vi "Status Update.vi"(8 "error in (no error)":errorcluster, 9 "Status":string, 10 "Name":string, 11 "Server in":refnum<class "Server.lvclass">) -> (0 "error out":errorcluster, 3 "Server out":refnum<class "Server.lvclass">)   [LabVIEW 2020, in "Server.lvlib" / "Server.lvclass"]
uses:
  Server.lvclass
  Server.lvclass/Server.ctl
  Chat Window Model/Chat Window Model Messages/Update Status Log Msg/Update Status Log Msg.lvclass/Update Status Log Msg.ctl
  <vilib>/ActorFramework/Message Enqueuer/Message Enqueuer.lvclass/Message Enqueuer.ctl
  <vilib>/ActorFramework/Message Enqueuer/Enqueue.vi
  Chat Window Model/Chat Window Model Messages/Update Status Log Msg/Update Status Log Msg.lvclass
  C:/Program Files/National Instruments/LabVIEW 2020/vi.lib/ActorFramework/Message/Message.lvclass
  <vilib>/ActorFramework/Message Priority Queue/Priority Enqueue.vi
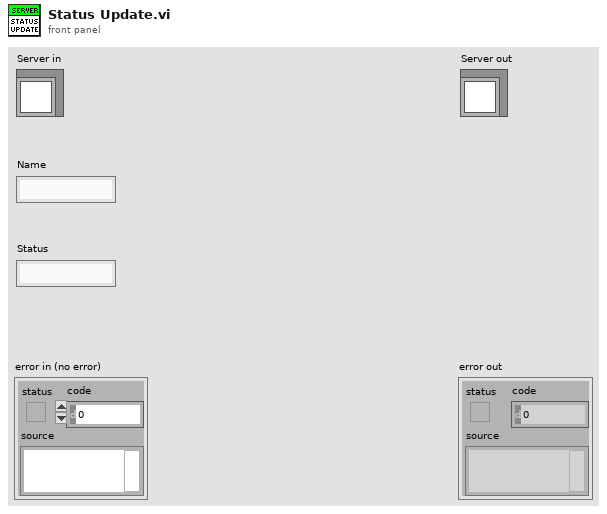
[diagram p1: front panel]
types:
  T1 = map{string, cluster{"Enqueuer":refnum<class "Message Enqueuer.lvclass">, "Status":string}}
  T2 = cluster{"Enqueuer":refnum<class "Message Enqueuer.lvclass">, "Status":string}
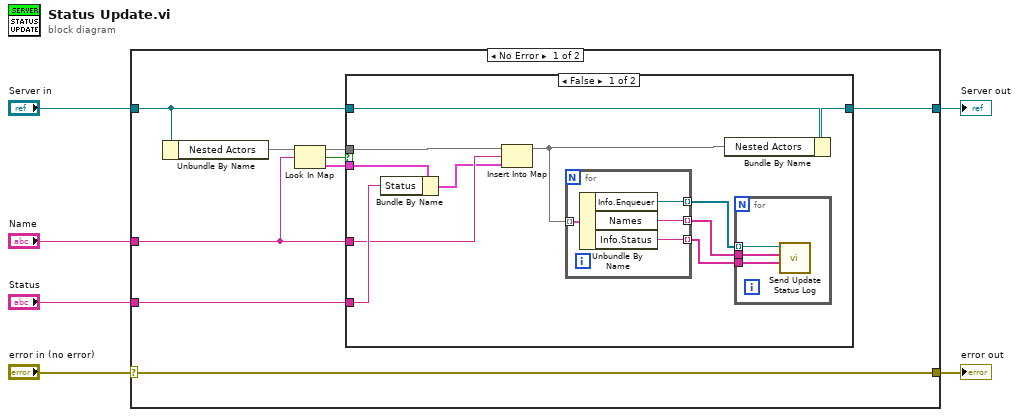
[diagram p0: block diagram]
diagram:
  n1 = case shown="No Error" "error in (no error)" {
    selector: "error in (no error)" -> [w14 w35]
    tunnel: [w14 w35] -> w5
    tunnel: [w12 w34] -> w3
    tunnel: "Server in" -> [w13 w34]
    tunnel: "Status" -> [w11 _]
    tunnel: "Name" -> [w7 _]
    frame No Error {
      n2 = Unbundle By Name(w13) -> ("Nested Actors"=w8:T1)
      n3 = Look In Map(map=w8, key=w7) -> (key not found?=w10:bool, value=w9:T2)  [unwired: 1 in]
      n4 = case shown="False" w10 {
        tunnel: w13 -> [w24 w33]
        tunnel: [w25 w33] -> w12
        tunnel: w11 -> [w22 _]
        tunnel: w9 -> [w23 _]
        tunnel: w8 -> [w21 _]
        tunnel: w7 -> [w20 _]
        frame False {
          n5 = Bundle By Name(cluster=w23, "Status"=w22) -> (w19:T2)
          n6 = Insert Into Map(map in=w21, key=w20, value=w19) -> (map out=w18:T1)  [unwired: 2 out]
          n7 = for {
            tunnel: w18 -> [w29] mode=indexing
            tunnel: [w28] -> w17 mode=indexing
            tunnel: [w27] -> w16 mode=indexing
            tunnel: [w26] -> w15 mode=indexing
            n8 = Unbundle By Name(w29) -> ("Info.Enqueuer"=w28:refnum<class "Message Enqueuer.lvclass">, "Names"=w27:string, "Info.Status"=w26:string)
          }
          n9 = Bundle By Name(cluster=w24, "Nested Actors"=w18) -> (w25:refnum<class "Server.lvclass">)
          n10 = for {
            tunnel: w15 -> [w31]
            tunnel: w17 -> [w32] mode=indexing
            tunnel: w16 -> [w30]
            n11 = call "Send Update Status Log.vi"("Status List"=w31, "Names"=w30, "Message Enqueuer"=w32) -> ()  [unwired: 7 in, 2 out]
          }
        }
        frame True {
        }
      }
    }
    frame Error {
    }
  }
  "error out" <- w5
  "Server out" <- w3
